vi "上升沿触发.vi"(1 "信号输入":i32) -> (0 "x与y?":bool)   [LabVIEW 2014]
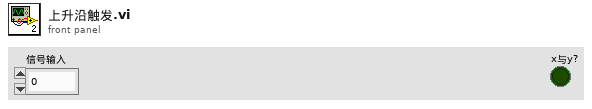
[diagram p1: front panel]
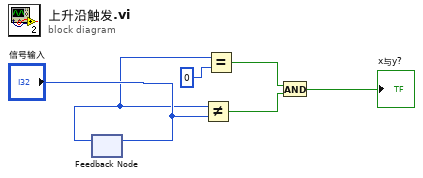
[diagram p0: block diagram]
diagram:
  n1 = feedback #1() -> (w1:i32)  [unwired: 1 in]
  n2 = feedback-in #1("信号输入") -> ()
  n3 = Not Equal?(x=w1, y="信号输入") -> (x != y?=w3:bool)
  n4 = Equal?(x=w1, y=0) -> (x = y?=w4:bool)
  n5 = And(x=w4, y=w3) -> (x .and. y?=→"x与y?":bool)
